vi "CMD_PowerSTEP01_GET_ABS_POS.vi"(8 "error in (no error)":errorcluster, 9 "write enable":bool=TRUE, 11 "SMSD in":refnum<class "SMSD Master.lvclass">) -> (0 "error out":errorcluster, 2 "position":i32, 3 "SMSD out":refnum<class "SMSD Master.lvclass">)   [LabVIEW 2021, in "SMSD Master.lvclass"]
uses:
  SMSD Master.lvclass
  Data Unit/SMSD Data Unit/ERROR_OR_COMMANT_Type.ctl
  Data Unit/SMSD Data Unit/SMSD Data Unit.lvclass/SMSD Data Unit.ctl
  SMSD Master.lvclass/SMSD Master.ctl
  Transmission Data Unit/SMSD/SMSD ADU.lvclass/SMSD ADU.ctl
  Devices/SMSD/SMSD_cmd_Data_format.vi
  Data Unit/SMSD Data Unit/Construct PDU.vi
  Read write Master.vi
  Data Unit/SMSD Data Unit/Deconstruct PDU.vi
  Transmission Data Unit/SMSD/Write ADU Packet.vi
  Transmission Data Unit/SMSD/Read ADU Packet.vi
  Modbus_v121c/Network Interface/TCP Interface/TCP Shared Components/TCP Write.vi
  Data Unit/SMSD Data Unit/Flatten PDU.vi
  Data Unit/SMSD Data Unit/Unflatten to PDU.vi
  Modbus_v121c/Network Interface/TCP Interface/TCP Shared Components/TCP Read.vi
  <vilib>/Utility/error.llb/Clear Errors.vi
  Data Unit/SMSD Data Unit/SMSD Data Unit.lvclass
  Devices/SMSD/SMSD.lvclass
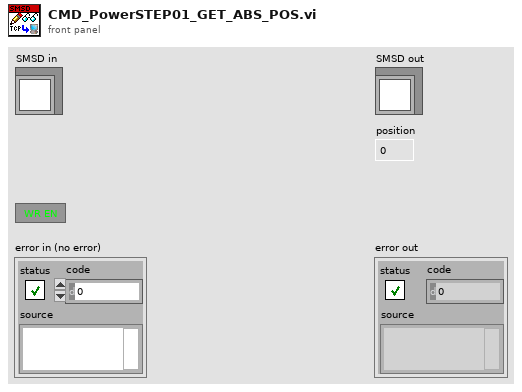
[diagram p1: front panel]
types:
  T1 = enum8{"CMD_PowerSTEP01_END", "CMD_PowerSTEP01_GET_SPEED", "CMD_PowerSTEP01_STATUS_IN_EVENT", "CMD_PowerSTEP01_SET_MODE", "CMD_PowerSTEP01_GET_MODE", "CMD_PowerSTEP01_SET_MIN_SPEED", "CMD_PowerSTEP01_SET_MAX_SPEED", "CMD_PowerSTEP01_SET_ACC", "CMD_PowerSTEP01_SET_DEC", "CMD_PowerSTEP01_SET_FS_SPEED", "CMD_PowerSTEP01_SET_MASK_EVENT", "CMD_PowerSTEP01_GET_ABS_POS", "CMD_PowerSTEP01_GET_EL_POS", "CMD_PowerSTEP01_GET_STATUS_AND_CLR", "CMD_PowerSTEP01_RUN_F", "CMD_PowerSTEP01_RUN_R", "CMD_PowerSTEP01_MOVE_F", "CMD_PowerSTEP01_MOVE_R", "CMD_PowerSTEP01_GO_TO_F", "CMD_PowerSTEP01_GO_TO_R", "CMD_PowerSTEP01_GO_UNTIL_F", "CMD_PowerSTEP01_GO_UNTIL_R", "CMD_PowerSTEP01_SCAN_ZERO_F", "CMD_PowerSTEP01_SCAN_ZERO_R", "CMD_PowerSTEP01_SCAN_LABEL_F", "CMD_PowerSTEP01_SCAN_LABEL_R", "CMD_PowerSTEP01_GO_ZERO", "CMD_PowerSTEP01_GO_LABEL", "CMD_PowerSTEP01_GO_TO", "CMD_PowerSTEP01_RESET_POS", "CMD_PowerSTEP01_RESET_POWERSTEP01", "CMD_PowerSTEP01_SOFT_STOP", "CMD_PowerSTEP01_HARD_STOP", "CMD_PowerSTEP01_SOFT_HI_Z", "CMD_PowerSTEP01_HARD_HI_Z", "CMD_PowerSTEP01_SET_WAIT", "CMD_PowerSTEP01_SET_RELE", "CMD_PowerSTEP01_CLR_RELE", "CMD_PowerSTEP01_GET_RELE", "CMD_PowerSTEP01_WAIT_IN0", "CMD_PowerSTEP01_WAIT_IN1", "CMD_PowerSTEP01_GOTO_PROGRAM", "CMD_PowerSTEP01_GOTO_PROGRAM_IF_IN0", "CMD_PowerSTEP01_GOTO_PROGRAM_IF_IN1", "CMD_PowerSTEP01_LOOP_PROGRAM", "CMD_PowerSTEP01_CALL_PROGRAM", "CMD_PowerSTEP01_RETURN_PROGRAM", "CMD_PowerSTEP01_START_PROGRAM_MEM0", "CMD_PowerSTEP01_START_PROGRAM_MEM1", "CMD_PowerSTEP01_START_PROGRAM_MEM2", "CMD_PowerSTEP01_START_PROGRAM_MEM3", "CMD_PowerSTEP01_STOP_PROGRAM_MEM", "CMD_PowerSTEP01_STEP_CLOCK", "CMD_PowerSTEP01_STOP_USB", "CMD_PowerSTEP01_GET_MIN_SPEED", "CMD_PowerSTEP01_GET_MAX_SPEED", "CMD_PowerSTEP01_GET_STACK", "CMD_PowerSTEP01_GOTO_PROGRAM_IF_ZERO", "CMD_PowerSTEP01_GOTO_PROGRAM_IF_IN_ZERO", "CMD_PowerSTEP01_WAIT_CONTINUE", "CMD_PowerSTEP01_SET_WAIT_2", "CMD_PowerSTEP01_SCAN_MARK2_F", "CMD_PowerSTEP01_SCAN_MARK2_R"}
  T2 = typedef "SMSD Data Unit.lvclass/ERROR_OR_COMMANT_Type.ctl" = enum8{"OK", "OK_ACCESS", "ERROR_ACCESS", "ERROR_ACCESS_TIMEOUT", "ERROR_XOR", "ERROR_NO_COMMAND", "ERROR_LEN", "ERROR_RANGE", "ERROR_WRITE", "ERROR_READ", "ERROR_PROGRAMS", "ERROR_WRITE_SETUP", "NO_NEXT", "END_PROGRAMS", "COMMAND_GET_STATUS_IN_EVENT", "COMMAND_GET_MODE", "COMMAND_GET_ABS_POS", "COMMAND_GET_EL_POS", "COMMAND_GET_SPEED", "COMMAND_GET_MIN_SPEED", "COMMAND_GET_MAX_SPEED", "COMMAND_GET_STACK", "STATUS_RELE_SET", "STATUS_RELE_CLR"}
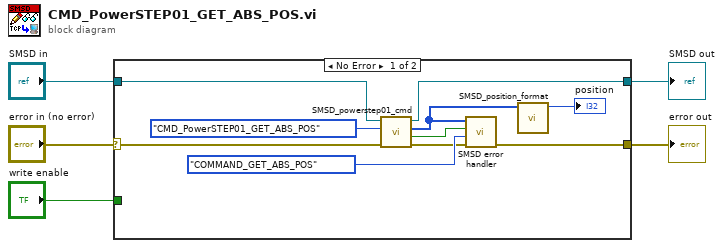
[diagram p0: block diagram]
diagram:
  n1 = case shown="No Error" "error in (no error)" {
    selector: "error in (no error)" -> [w9 w17]
    tunnel: [w6 w17] -> w1
    tunnel: [w7 w16] -> w2
    tunnel: "SMSD in" -> [w8 w16]
    tunnel: "write enable" -> [_ _]
    frame No Error {
      n2 = call "SMSD_powerstep01_cmd.vi"("error in (no error)"=w9, "COMMAND (END)"=T1."CMD_PowerSTEP01_GET_ABS_POS", "SMSD in"=w8) -> ("error out"=w13:errorcluster, "PDU valid?"=w11:bool, "data"=w14:u8[], "SMSD out"=w7:refnum<class "SMSD Master.lvclass">)  [unwired: 5 in]
      n3 = call "SMSD error handler.vi"("error in (no error)"=w13, "correct answer (OK)"=ERROR_OR_COMMANT_Type."COMMAND_GET_ABS_POS" ("coerced x 2"), "timed out?"=w11, "data"=w14) -> ("error out"=w6:errorcluster)  [unwired: 7 in]
      n4 = call "SMSD_position_format.vi"("DATA"=w14) -> ("position"=→"position":i32)  [unwired: 10 in]
    }
    frame Error {
    }
  }
  "error out" <- w1
  "SMSD out" <- w2
